vi "SekwencjaFZG.vi"() -> ()   [LabVIEW 2024]
uses:
  FZG.ctl
panel:
  out "Wyjœcie":dbl
  in  "Wejœcie":dbl
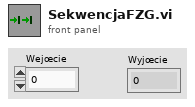
[diagram p1: front panel]
types:
  T1 = typedef "FZG.ctl" = enum16{"Clear", "AddElement", "SubElement", "MulElement", "DivElement", "PowElement"}
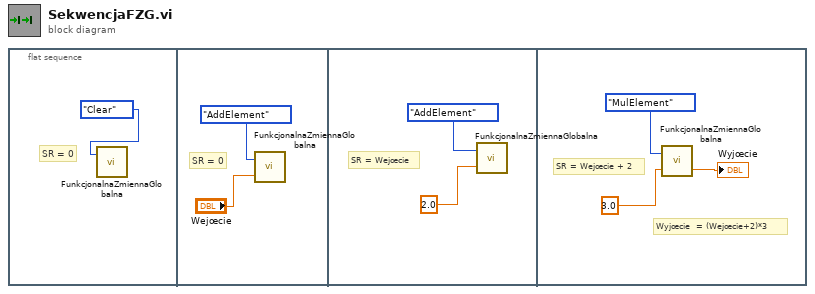
[diagram p0: block diagram]
diagram:
  n1 = flat-sequence {
    frame #0 {
      # "SR = 0"
      n2 = call "FunkcjonalnaZmiennaGlobalna.vi"("Stan"=FZG."Clear") -> ()  [unwired: 2 in, 1 out]
    }
    frame #1 {
      # "SR = 0"
      n3 = call "FunkcjonalnaZmiennaGlobalna.vi"("Wejœcie"="Wejœcie", "Stan"=FZG."AddElement") -> ()  [unwired: 1 in, 1 out]
    }
    frame #2 {
      # "SR = Wejœcie"
      n4 = call "FunkcjonalnaZmiennaGlobalna.vi"("Wejœcie"=2.0, "Stan"=FZG."AddElement") -> ()  [unwired: 1 in, 1 out]
    }
    frame #3 {
      # "Wyjœcie  = (Wejœcie+2)*3"
      # "SR = Wejœcie + 2"
      n5 = call "FunkcjonalnaZmiennaGlobalna.vi"("Wejœcie"=3.0, "Stan"=FZG."MulElement") -> ("Wyjœcie"=→"Wyjœcie":dbl)  [unwired: 1 in]
    }
  }
